vi "CRYUnit-dBref std string parse.vi"(7 "Linear data":bool, 11 "Std. header string in":string) -> (1 "dB ref":dbl format="%.2f", 2 "Unit":string, 3 "Prefix":string)   [LabVIEW 2013]
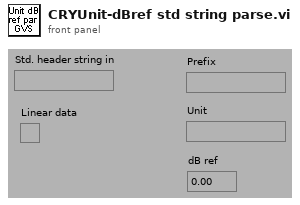
[diagram p1: front panel]
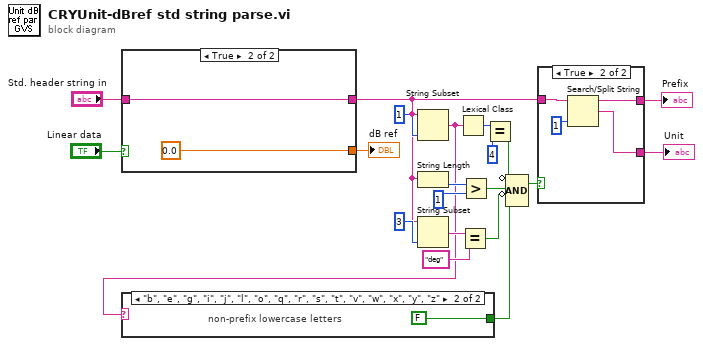
[diagram p0: block diagram]
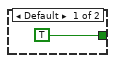
[diagram p2: hidden frame]
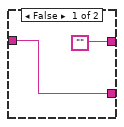
[diagram p3: hidden frame]
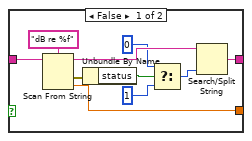
[diagram p4: hidden frame]
diagram:
  n1 = case shown="True" "Linear data" {
    tunnel: "Std. header string in" -> [w28 w32]
    tunnel: [w27 w32] -> w6
    tunnel: [w26 0.0] -> w18
    frame False {
      n2 = Scan From String(format string="dB re %f", input string=w28) -> (remaining string=w29:string, error out=w25:errorcluster, output 1=w26:dbl)  [unwired: 2 in, 2 out]
      n3 = Unbundle By Name(w25) -> ("status"=w24:bool)
      n4 = Select(t=0 ("offset (0)"), s=w24, f=1 ("offset (0)")) -> (s? t:f=w21:i32)
      n5 = Search/Split String(string=w29, offset (0)=w21) -> (match + rest of string=w27:string)  [unwired: 3 out]
    }
    frame True {
    }
  }
  "dB ref" <- w18
  n6 = String Subset(string=w6, length (rest)=1 ("length")) -> (substring=w2:string)  [unwired: 1 out]
  n7 = case shown="\"b\", \"e\", \"g\", \"i\", \"j\", \"l\", \"o\", \"q\", \"r\", \"s\", \"t\", \"v\", \"w\", \"x\", \"y\", \"z\"" w2 {
    tunnel: [TRUE FALSE] -> w1
    frame Default {
    }
    frame "b", "e", "g", "i", "j", "l", "o", "q", "r", "s", "t", "v", "w", "x", "y", "z" {
      # "non-prefix lowercase letters"
    }
  }
  n8 = String Length(string=w6) -> (length=w16:i32)
  n9 = String Subset(string=w6, length (rest)=3 ("length")) -> (substring=w5:string)  [unwired: 1 out]
  n10 = Lexical Class(1:w2) -> (0:w14:i16)
  n11 = Equal?(x=w5, y="deg") -> (x = y?=w3:bool)
  n12 = Greater?(x=w16, y=1) -> (0:w12:bool)
  n13 = Equal?(x=w14, y=i16 4) -> (x = y?=w11:bool)
  n14 = Compound Arithmetic op=AND(invert w11, w12, invert w3, w1) -> (w10:bool)
  n15 = case shown="True" w10 {
    tunnel: w6 -> [w35 w37]
    tunnel: ["" w39] -> w9
    tunnel: [w35 w38] -> w8
    frame False {
    }
    frame True {
      n16 = Search/Split String(string=w37, offset (0)=1) -> (substring before match=w39:string, match + rest of string=w38:string)  [unwired: 2 out]
    }
  }
  "Prefix" <- w9
  "Unit" <- w8
